vi "Remote Client.vi"(5 "Port":u16=6341, 6 "Wait for Response?":bool, 7 "address":string, 8 "error in (no error)":errorcluster, 9 "Data":variant, 10 "Command":string, 11 "RemoteControl in":refnum<class "RemoteControl.lvclass">) -> (0 "error out":errorcluster, 1 "Data out":variant, 2 "Command out":string, 3 "RemoteControl out":refnum<class "RemoteControl.lvclass">)   [LabVIEW 2016, in "RemoteControl.lvclass"]
uses:
  RemoteControl.lvclass
panel:
  out "execution time (ms)":u32
  # "Simple Client"
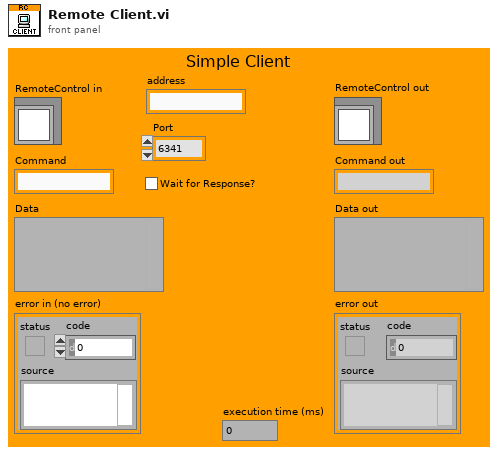
[diagram p1: front panel]
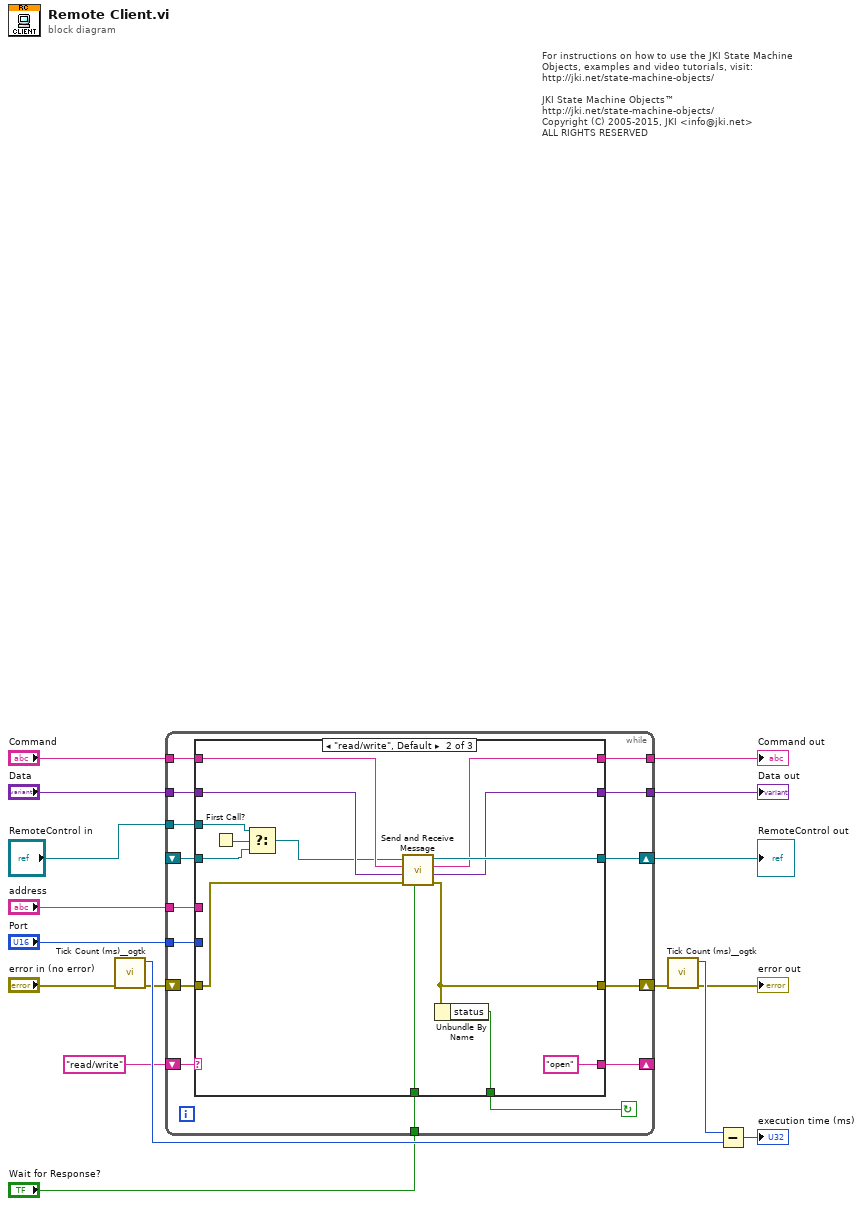
[diagram p0: block diagram]
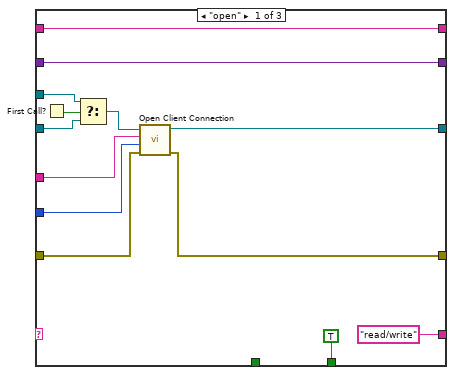
[diagram p2: hidden frame]
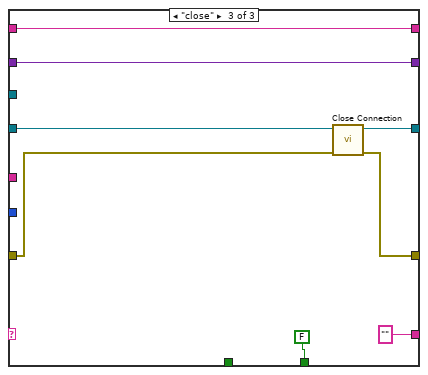
[diagram p3: hidden frame]
diagram:
  # "For instructions on how to use the JKI State Machine Objects, examples and video tutorials, visit:\nhttp://jki.net/state-machine-objects/\n\nJKI State Machine Objects™\nhttp://jki.net/state-machine-objects/\nCopyright (C) 2005-2015, JKI <info@jki.net>\nALL RIGHTS RESERVED"
  n1 = call <userlib>:"Tick Count (ms)__ogtk.vi"("error in (no error)"="error in (no error)") -> ("error out"=w9:errorcluster, "millisecond timer value"=w14:u32)  [unwired: 9 in]
  n2 = while {
    tunnel: "Port" -> [w30]
    tunnel: "address" -> [w28]
    tunnel: "Wait for Response?" -> [w27]
    shift-right: [w31] -> w12
    shift-left: w9 -> [w29]
    shift-right: [w32] -> w13
    shift-left: _ -> [w18]
    shift-right: [w21] -> _
    shift-left: "read/write" -> [w22]
    tunnel: "RemoteControl in" -> [w19]
    tunnel: "Data" -> [w26]
    tunnel: [w23] -> w3
    tunnel: "Command" -> [w25]
    tunnel: [w24] -> w4
    stop <- w20 continue-if-true
    n3 = case shown="\"read/write\", Default" w22 {
      tunnel: [w42 w55 w67] -> w32
      tunnel: [w41 w47 w66] -> w31
      tunnel: w30 -> [w45 _ _]
      tunnel: w29 -> [w44 w59 w65]
      tunnel: w18 -> [w35 w50 w64]
      tunnel: w28 -> [w43 _ _]
      tunnel: w27 -> [_ w58 _]
      tunnel: w26 -> [w40 w57 w63]
      tunnel: w25 -> [w39 w56 w62]
      tunnel: [w39 w54 w62] -> w24
      tunnel: [w40 w53 w63] -> w23
      tunnel: ["read/write" "open" ""] -> w21
      tunnel: [TRUE w46 FALSE] -> w20
      tunnel: w19 -> [w33 w49 _]
      frame "open" {
        n4 = First Call?() -> (First Call?: T/F=w36:bool)
        n5 = Select(t=w33, s=w36, f=w35) -> (s? t:f=w34:refnum<class "RemoteControl.lvclass">)
        n6 = call-dynamic "Open Client Connection.vi"("error in (no error)"=w44, "Port"=w45, "address"=w43, "RemoteControl in"=w34) -> ("error out"=w41:errorcluster, "RemoteControl out"=w42:refnum<class "RemoteControl.lvclass">)  [unwired: 6 in]
      }
      frame "read/write", Default {
        n7 = First Call?() -> (First Call?: T/F=w51:bool)
        n8 = Select(t=w49, s=w51, f=w50) -> (s? t:f=w48:refnum<class "RemoteControl.lvclass">)
        n9 = call-dynamic "Send and Receive Message.vi"("Wait for response?"=w58, "error in (no error)"=w59, "Data"=w57, "Command"=w56, "RemoteControl in"=w48) -> ("error out"=w47:errorcluster, "Data out"=w53:variant, "Command out"=w54:string, "RemoteControl out"=w55:refnum<class "RemoteControl.lvclass">)  [unwired: 3 in]
        n10 = Unbundle By Name(w47) -> ("status"=w46:bool)
      }
      frame "close" {
        n11 = call-dynamic "Close Connection.vi"("error in (no error)"=w65, "RemoteControl in"=w64) -> ("error out"=w66:errorcluster, "RemoteControl out"=w67:refnum<class "RemoteControl.lvclass">)  [unwired: 8 in]
      }
    }
  }
  "RemoteControl out" <- w13
  "Data out" <- w3
  "Command out" <- w4
  n12 = call <userlib>:"Tick Count (ms)__ogtk.vi"("error in (no error)"=w12) -> ("error out"=→"error out":errorcluster, "millisecond timer value"=w17:u32)  [unwired: 9 in]
  n13 = Subtract(x=w17, y=w14) -> (x-y=→"execution time (ms)":u32)
